vi "Mouse Up.vi"(8 "error in (no error)":errorcluster, 10 "Point":T1, 11 "Geometric Object in":refnum<class "Graphics Object.lvclass">) -> (0 "error out":errorcluster, 3 "Geometric Object out":refnum<class "Graphics Object.lvclass">)   [LabVIEW 2018, in "Graphics Object.lvclass"]
doc: "A method for specifying how a graphics object reacts on a mouse up event."
uses:
  Graphics Object.lvclass
  <vilib>/Utility/miscctls.llb/LVPoint32TypeDef.ctl
  Graphics Object.lvclass/Graphics Object.ctl
panel:
  # "expressionflow.com"
  # "Copyright (c) 2008 Tomi Maila. All rights reserved."
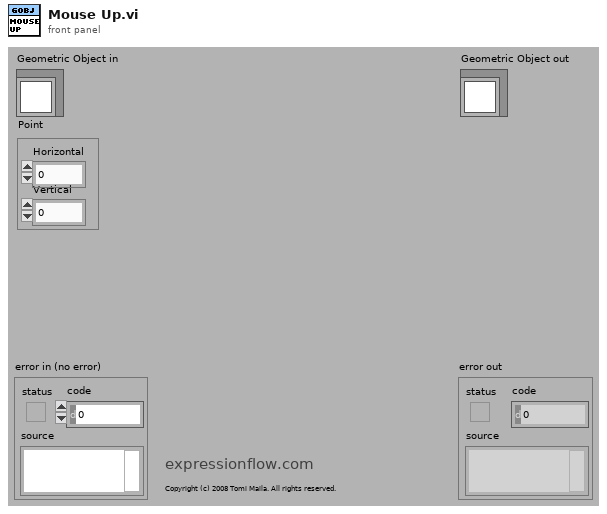
[diagram p1: front panel]
types:
  T1 = typedef "LVPoint32TypeDef.ctl" = cluster{"Horizontal":i32, "Vertical":i32}
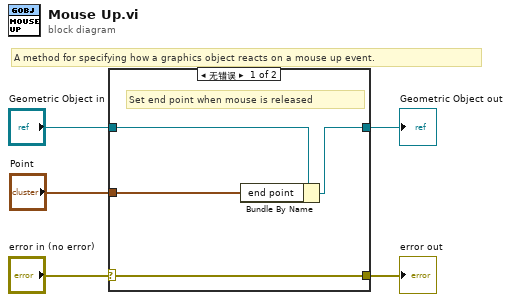
[diagram p0: block diagram]
diagram:
  # "A method for specifying how a graphics object reacts on a mouse up event."
  n1 = case shown="无错误" "error in (no error)" {
    selector: "error in (no error)" -> [w9 w10]
    tunnel: [w9 w10] -> w1
    tunnel: [w7 w11] -> w4
    tunnel: "Geometric Object in" -> [w8 w11]
    tunnel: "Point" -> [w6 _]
    frame No Error {
      # "Set end point when mouse is released"
      n2 = Bundle By Name(cluster=w8, "end point"=w6) -> (w7:refnum<class "Graphics Object.lvclass">)
    }
    frame Error {
    }
  }
  "error out" <- w1
  "Geometric Object out" <- w4
